vi "Line_name_string.vi"(7 "Type":string="Front valve ", 9 "i":i32) -> (1 "name out":string)   [LabVIEW 2016]
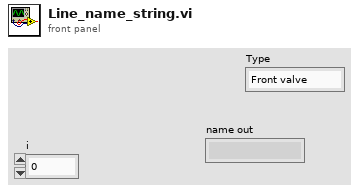
[diagram p1: front panel]
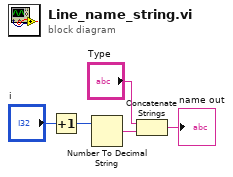
[diagram p0: block diagram]
diagram:
  n1 = Increment(x="i") -> (x+1=w1:i32)
  n2 = Number To Decimal String(number=w1) -> (decimal integer string=w2:string)  [unwired: 1 in]
  n3 = Concatenate Strings("Type", w2) -> (→"name out":string)
